vi "compute_jula_set.vi"(6 "x + iy":cdb, 7 "max iter":i32=100, 10 "y axis":T1={"samples"=1000, "end"=1.0, "start"=-1.0}, 11 "x axis":T1={"samples"=1000, "end"=1.0, "start"=-1.0}) -> (2 "render time":dbl, 3 "fractal set":i32[][](graph))   [LabVIEW 2019, in "Mandelbrot.lvlib"]
uses:
  Mandelbrot.lvlib
  axis_info.ctl
  <vilib>/Analysis/1siggen.llb/Ramp Pattern by Samples.vi
  <vilib>/Analysis/NI_AALBase.lvlib
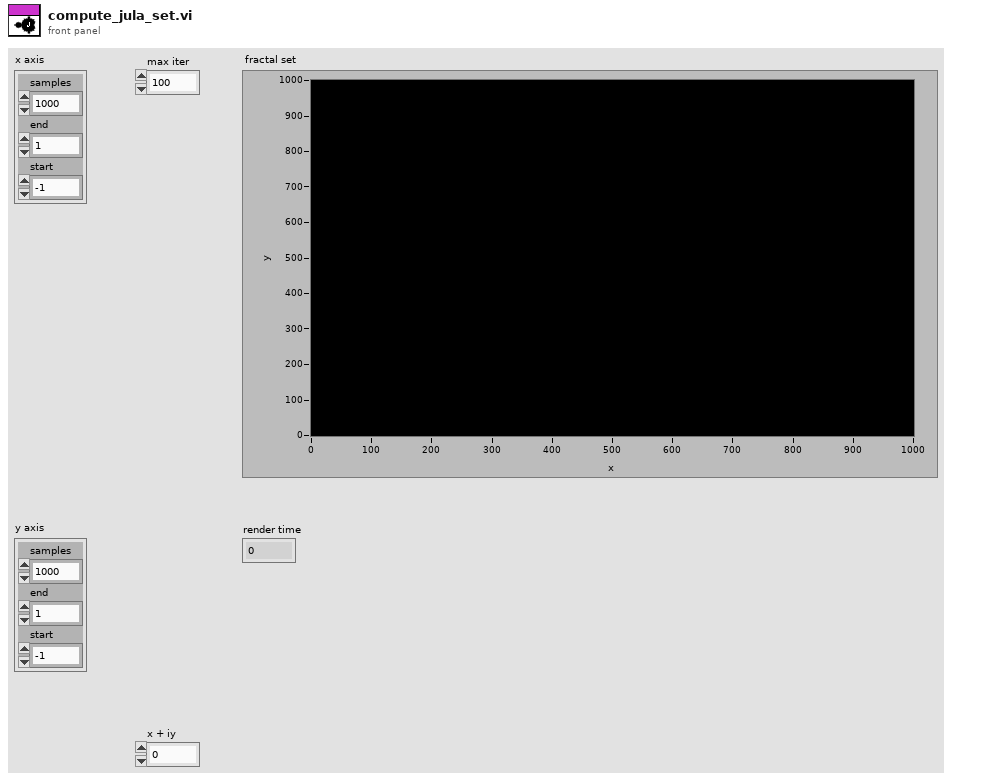
[diagram p1: front panel]
types:
  T1 = typedef "Mandelbrot.lvlib/axis_info.ctl" = cluster{"samples":u32, "end":dbl, "start":dbl}
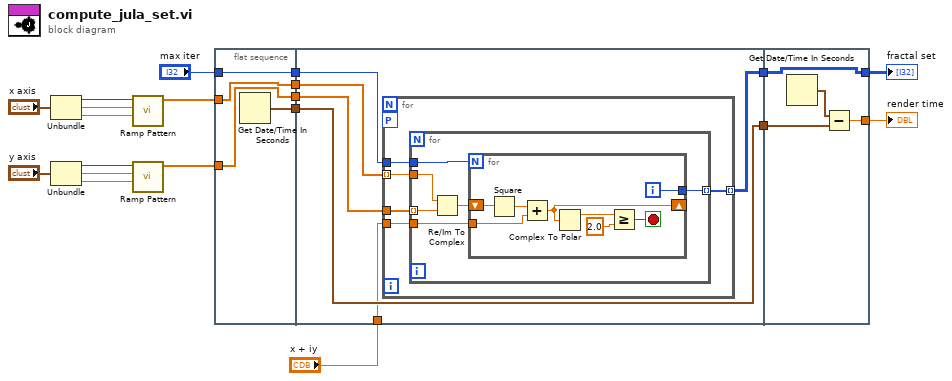
[diagram p0: block diagram]
diagram:
  n1 = Unbundle("x axis") -> ("samples"=w19:u32, "end"=w18:dbl, "start"=w17:dbl)
  n2 = Unbundle("y axis") -> ("samples"=w15:u32, "end"=w14:dbl, "start"=w13:dbl)
  n3 = call-poly <vilib>:"Ramp Pattern.vi"("start"=w17, "end"=w18, "samples"=w19) -> ("Ramp Pattern"=w11:dbl[])  [unwired: 7 in, 1 out]
  n4 = call-poly <vilib>:"Ramp Pattern.vi"("start"=w13, "end"=w14, "samples"=w15) -> ("Ramp Pattern"=w10:dbl[])  [unwired: 7 in, 1 out]
  n5 = flat-sequence {
    tunnel: w10 -> [w22]
    tunnel: w11 -> [w23]
    tunnel: "max iter" -> [w24]
    tunnel: [w24] -> w7
    tunnel: [w23] -> w6
    tunnel: [w22] -> w5
    tunnel: [w21] -> w4
    tunnel: [w27] -> w8
    tunnel: w7 -> [w30]
    tunnel: w6 -> [w29]
    tunnel: w5 -> [w28]
    tunnel: w4 -> [w26]
    tunnel: [w26] -> w3
    tunnel: "x + iy" -> [w25]
    tunnel: [w53] -> w9
    tunnel: w8 -> [w53]
    tunnel: w3 -> [w51]
    tunnel: [w50] -> w2
    frame #0 {
      n6 = Get Date/Time In Seconds() -> (seconds since 1Jan1904=w21:timestamp)
    }
    frame #1 {
      n7 = for {
        tunnel: w30 -> [w35]
        tunnel: w29 -> [w34] mode=indexing
        tunnel: w28 -> [w33]
        tunnel: [w32] -> w27 mode=indexing
        workers-P: _ -> [_]
        tunnel: w25 -> [w31]
        n8 = for {
          tunnel: w35 -> [w41]
          tunnel: w34 -> [w40]
          tunnel: w33 -> [w39] mode=indexing
          tunnel: [w38] -> w32 mode=indexing
          tunnel: w31 -> [w36]
          n9 = Re/Im To Complex(1:w39, 2:w40) -> (0:w37:cdb)
          n10 = for {
            N: w41 -> [_]
            shift-right: [w44] -> _
            shift-left: w37 -> [w49]
            tunnel: w36 -> [w47]
            tunnel: [w42] -> w38
            i -> [w42]
            stop <- w43 stop-if-true
            n11 = Square(x=w49) -> (x^2=w48:cdb)
            n12 = Add(x=w48, y=w47) -> (x+y=w44:cdb)
            n13 = Complex To Polar(r * e^(i*theta)=w44) -> (r=w46:dbl)  [unwired: 1 out]
            n14 = Greater Or Equal?(x=w46, y=2.0) -> (x >= y?=w43:bool)
          }
        }
      }
    }
    frame #2 {
      n15 = Get Date/Time In Seconds() -> (seconds since 1Jan1904=w52:timestamp)
      n16 = Subtract(x=w52, y=w51) -> (x-y=w50:dbl)
    }
  }
  "fractal set" <- w9
  "render time" <- w2
